vi "CAN Jaguar Set Transaction.vi"(8 "error in":errorcluster, 9 "Data":u8[](array[numeric]), 10 "Message ID":u32, 11 "CAN Jaguar Ref":T1={"Device Number"=0, "Control Mode"=enum."Percent VBus", "Inverted"=FALSE, "Semaphore"=refnum, "Max Vout"=12.0, "DevStatus"={"status"=FALSE, "code"=0, "source"=""}}) -> (0 "error out":errorcluster, 3 "CAN Jaguar Ref Out":T1={"Device Number"=0, "Control Mode"=enum."Percent VBus", "Inverted"=FALSE, "Semaphore"=refnum, "Max Vout"=12.0, "DevStatus"={"status"=FALSE, "code"=0, "source"=""}})   [LabVIEW 2009, in "CAN.lvlib"]
uses:
  CAN.lvlib
  CAN Jaguar Ref.ctl
  CAN Jaguar Control Mode.ctl
  CAN Motor Message IDs.ctl
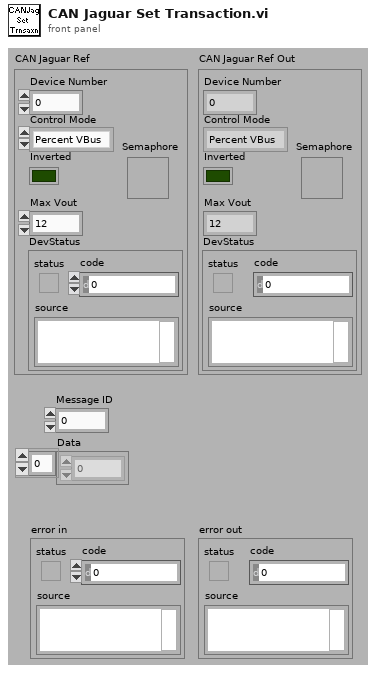
[diagram p1: front panel]
types:
  T1 = typedef "CAN.lvlib/CAN Jaguar Ref.ctl" = cluster{"Device Number":u8, "Control Mode":T2, "Inverted":bool, "Semaphore":T3, "Max Vout":dbl, "DevStatus":errorcluster}
  T2 = typedef "CAN.lvlib/CAN Jaguar Control Mode.ctl" = enum16{"Percent VBus", "Speed", "Position", "Current"}
  T3 = typedef "Semaphore RefNum" = refnum<k1>
  T4 = typedef "CAN.lvlib/CAN Motor Message IDs.ctl" = u32
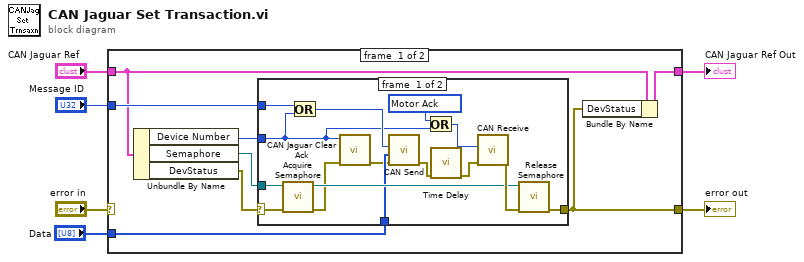
[diagram p0: block diagram]
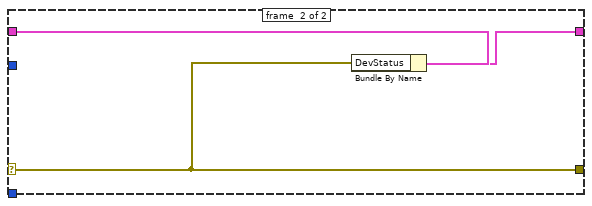
[diagram p3: hidden frame]
diagram:
  n1 = case shown="No Error" "error in" {
    selector: "error in" -> [_ w31]
    tunnel: "Message ID" -> [w14 _]
    tunnel: [w10 w31] -> w5
    tunnel: "CAN Jaguar Ref" -> [w12 w33]
    tunnel: [w11 w32] -> w2
    tunnel: "Data" -> [w9 _]
    frame #0 {
      n2 = Unbundle By Name(w12) -> ("Device Number"=w8:u8, "Semaphore"=w13:T3, "DevStatus"=w7:errorcluster)
      n3 = case shown="No Error" w7 {
        selector: w7 -> [w17 w30]
        tunnel: w14 -> [w29 _]
        tunnel: w13 -> [w27 _]
        tunnel: [w25 w30] -> w10
        tunnel: w9 -> [w23 _]
        tunnel: w8 -> [w18 _]
        frame #0 {
          w21 = T4 33693696 items=["Volt Enable"=33685504, "Volt Disable"=33685568, "Volt Set"=33685632, "Volt Set Ramp"=33685696, "Speed Enable"=33686528, "Speed Disable"=33686592, "Speed Set"=33686656, "Speed P"=33686720, "Speed I"=33686784, "Speed D"=33686848, "Speed Ref"=33686912, "Position Enable"=33688576, "Position Disable"=33688640, "Position Set"=33688704, "Position P"=33688768, "Position I"=33688832, "Position D"=33688896, "Position Ref"=33688960, "Current Enable"=33689600, "Current Disable"=33689664, "Current Set"=33689728, "Current P"=33689792, "Current I"=33689856, "Current D"=33689920, "Status VOut"=33690624, "Status VBus"=33690688, "Status Current"=33690752, "Status Temp"=33690816, "Status Position"=33690880, "Status Speed"=33690944, "Status Limit"=33691008, "Status Fault"=33691072, "Status Power"=33691136, "Config Num Brushes"=33692672, "Config Encoder Lines"=33692736, "Config Pot Turns"=33692800, "Config Brake Coast"=33692864, "Config Limit Mode"=33692928, "Config Limit Fwd"=33692992, "Config Limit Rev"=33693056, "Config Max VOut"=33693120, "Config Fault Time"=33693184, "Motor Ack"=33693696] ("CAN Motor Message IDs")
          n4 = call <vilib>:"Acquire Semaphore.vi"("error in (no error)"=w17, "semaphore"=w27) -> ("error out"=w20:errorcluster, "semaphore out"=w24:T3)  [unwired: 1 in, 3 out]
          n5 = Or(x=w29, y=w18) -> (x .or. y?=w28:u32)
          n6 = call "CAN Jaguar Clear Ack.vi"("DevStatus"=w20, "Device Number"=w18) -> ("error out"=w19:errorcluster)  [unwired: 9 out]
          n7 = call "CAN Send.vi"("error in (no error)"=w19, "data"=w23, "messageID"=w28) -> ("error out"=w15:errorcluster)  [unwired: 8 out]
          n8 = Or(x=w21, y=w18) -> (x .or. y?=w22:T4)
          n9 = call "Time Delay"("error in (no error)"=w15) -> ("error out"=w16:errorcluster)  [unwired: 10 in]
          n10 = call "CAN Receive.vi"("error in (no error)"=w16, "Message ID"=w22) -> ("error out"=w26:errorcluster)  [unwired: 1 in, 8 out]
          n11 = call <vilib>:"Release Semaphore.vi"("error in (no error)"=w26, "semaphore"=w24) -> ("error out"=w25:errorcluster)  [unwired: 5 out]
        }
        frame #1 {
        }
      }
      n12 = Bundle By Name(cluster=w12, "DevStatus"=w10) -> (w11:T1)
    }
    frame #1 {
      n13 = Bundle By Name(cluster=w33, "DevStatus"=w31) -> (w32:T1)
    }
  }
  "error out" <- w5
  "CAN Jaguar Ref Out" <- w2
